vi "Get Button.vi"(8 "error in (no error)":errorcluster, 11 "MouseEventArgs in":refnum<class "MouseEventArgs.lvclass">) -> (0 "error out":errorcluster, 2 "Button":i32(ring) items=["None"=0, "Left"=1048576, "Right"=2097152, "Middle"=4194304, "XButton1"=8388608, "XButton2"=16777216], 3 "MouseEventArgs out":refnum<class "MouseEventArgs.lvclass">)   [LabVIEW 2023, in "SourceGrid.lvlib" / "MouseEventArgs.lvclass"]
doc: "Gets which mouse button was pressed."
uses:
  MouseEventArgs.lvclass
  MouseEventArgs.lvclass/MouseEventArgs.ctl
  System.Windows.Forms
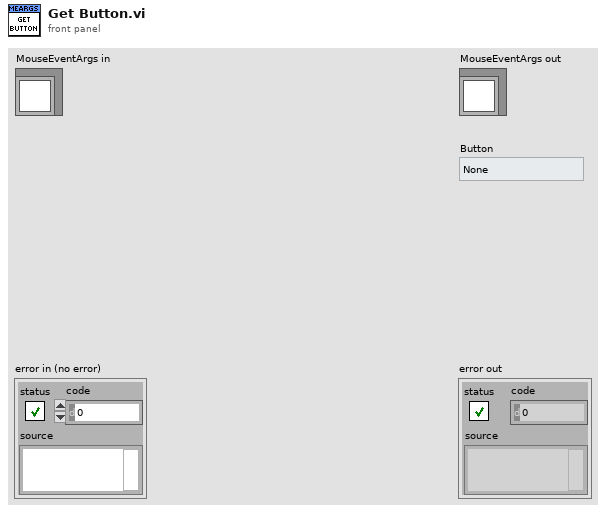
[diagram p1: front panel]
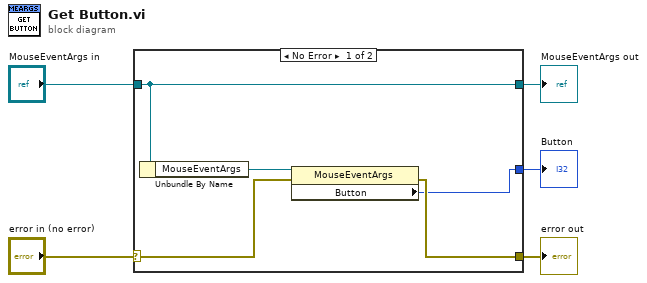
[diagram p0: block diagram]
diagram:
  n1 = case shown="No Error" "error in (no error)" {
    selector: "error in (no error)" -> [w8 w11]
    tunnel: [w7 w11] -> w4
    tunnel: [w10 w12] -> w2
    tunnel: "MouseEventArgs in" -> [w10 w12]
    tunnel: [w6 _] -> w1
    frame No Error {
      n2 = Unbundle By Name(w10) -> ("MouseEventArgs"=w9:refnum<k24>)
      n3 = property class="MouseEventArgs"(reference=w9, error in=w8) -> (error out=w7:errorcluster, "Button"=w6:i32)  [unwired: 1 out]
    }
    frame Error {
    }
  }
  "error out" <- w4
  "MouseEventArgs out" <- w2
  "Button" <- w1
